vi "Read XY Stage Controller.vi"(8 "error in (no error)":errorcluster, 11 "In":refnum<class "XY Stage Class.lvclass">) -> (0 "error out":errorcluster, 2 "XY Stage Controller":refnum<class "XY Stage Controller.lvclass">, 3 "Out":refnum<class "XY Stage Class.lvclass">)   [LabVIEW 2022 SP3, in "XY Stage Class.lvclass"]
uses:
  XY Stage Class.lvclass
  XY Stage Class.lvclass/XY Stage Class.ctl
  XY Controller/XY Stage Controller/XY Stage Controller.lvclass
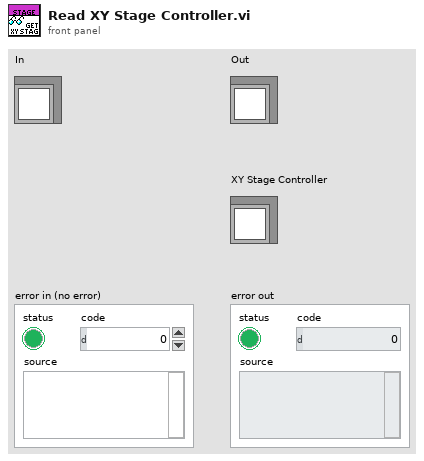
[diagram p1: front panel]
types:
  T1 = typedef "XY Stage Class.lvclass/data.ctl" = cluster{"XY Stage Controller":refnum<class "XY Stage Controller.lvclass">}
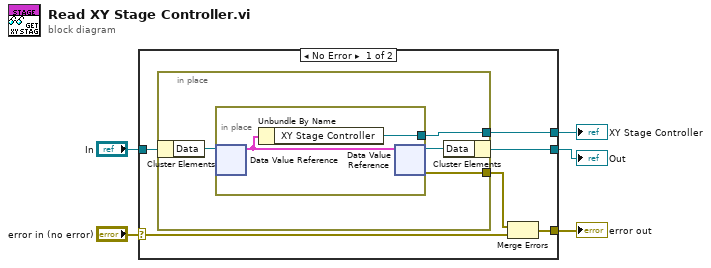
[diagram p0: block diagram]
diagram:
  n1 = case shown="No Error" "error in (no error)" {
    selector: "error in (no error)" -> [w6 w19]
    tunnel: [w7 w19] -> w4
    tunnel: [w11 w18] -> w3
    tunnel: "In" -> [w10 w18]
    tunnel: [w9 _] -> w1
    frame No Error {
      n2 = in-place {
        in-place-border: [w13] -> w9
        in-place-border: [w12] -> w8
        n3 = in-place-cluster #1(w10) -> ("Data"=w14:refnum<data-value>)
        n4 = in-place {
          in-place-border: [w16] -> w13
          n5 = in-place-dvr #2(w14) -> (w17:T1)  [unwired: 1 out]
          n6 = Unbundle By Name(w17) -> ("XY Stage Controller"=w16:refnum<class "XY Stage Controller.lvclass">)
          n7 = in-place-dvr #2(w17) -> (w15:refnum<data-value>, w12:errorcluster)
        }
        n8 = in-place-cluster #1("Data"=w15) -> (w11:refnum<class "XY Stage Class.lvclass">)
      }
      n9 = Merge Errors(w8, w6) -> (w7:errorcluster)
    }
    frame Error {
    }
  }
  "Out" <- w3
  "error out" <- w4
  "XY Stage Controller" <- w1
